vi "2. Термометр.vi"() -> ()   [LabVIEW 2020]
panel:
  in  "Максимально допустимое значение \nтемпературы в градусах Реамюра, R":dbl
  out "String":string
  out "Количества выполненных измерений температуры":i32
  out "Выходное напряжение \nдатчика температуры, В":dbl(knob) scale=0.0..23.0
  out "Текущее значение температуры \nв градусах Реамюра, R":dbl
  out "Текущее значение температуры\nв градусах Фаренгейта, F":dbl
  out "Температура в градусах Реамюра, R":dbl(slide) scale=0.0..21.0
  out "Температура в градусах Фаренгейта, F":dbl(slide) scale=0.0..78.0
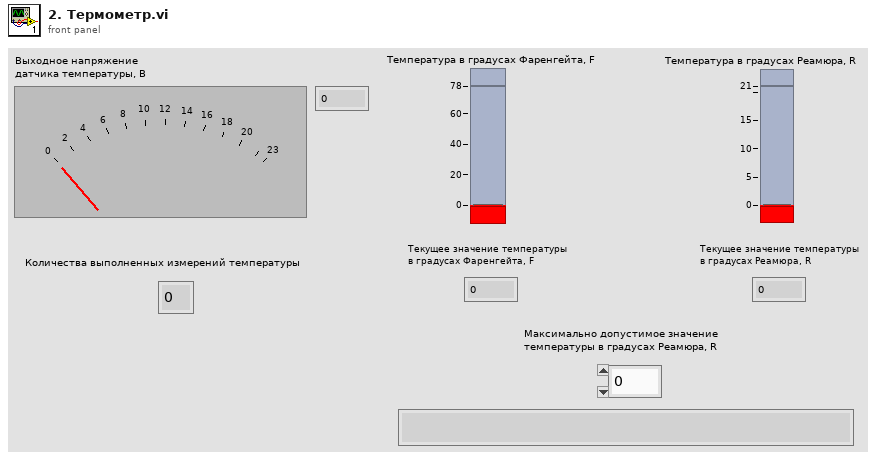
[diagram p1: front panel]
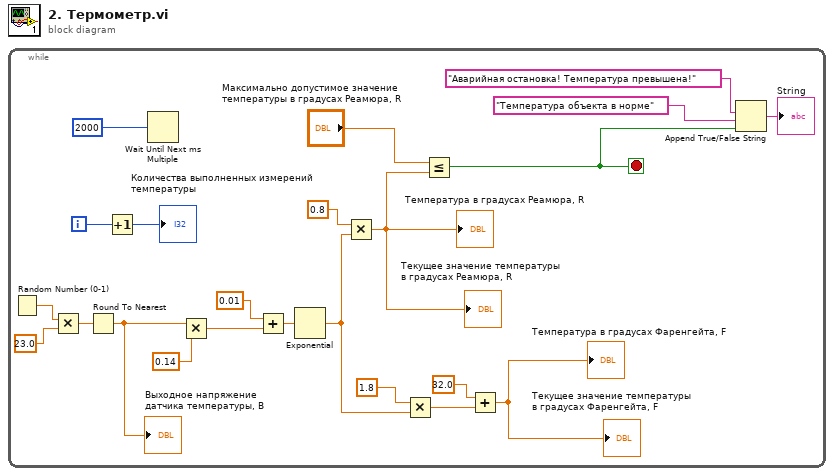
[diagram p0: block diagram]
diagram:
  n1 = while {
    i -> [w8]
    stop <- w4 stop-if-true
    n2 = Random Number (0-1)() -> (number: 0 to 1=w18:dbl)
    n3 = Multiply(x=w18, y=23.0) -> (x*y=w19:dbl)
    n4 = Round To Nearest(number=w19) -> (nearest integer value=w20:dbl)
    "Выходное напряжение \nдатчика температуры, В" <- w20
    n5 = Increment(x=w8) -> (x+1=→"Количества выполненных измерений температуры":i32)
    n6 = Wait Until Next ms Multiple(millisecond multiple=u32 2000 ("millisecond timer value")) -> ()  [unwired: 1 out]
    n7 = Multiply(x=w20, y=0.14) -> (x*y=w15:dbl)
    n8 = Add(x=0.01, y=w15) -> (x+y=w16:dbl)
    n9 = Exponential(1:w16) -> (0:w21:dbl)
    n10 = Multiply(x=0.8, y=w21) -> (x*y=w3:dbl)
    "Температура в градусах Реамюра, R" <- w3
    "Текущее значение температуры \nв градусах Реамюра, R" <- w3
    n11 = Multiply(x=1.8, y=w21) -> (x*y=w17:dbl)
    n12 = Less Or Equal?(x="Максимально допустимое значение \nтемпературы в градусах Реамюра, R", y=w3) -> (x <= y?=w4:bool)
    n13 = Add(x=32.0, y=w17) -> (x+y=→"Температура в градусах Фаренгейта, F" →"Текущее значение температуры\nв градусах Фаренгейта, F":dbl)
    n14 = Append True/False String(1:w4, 2:"Температура объекта в норме", 3:"Аварийная остановка! Температура превышена!") -> (0:→"String":string)  [unwired: 1 in]
  }
